vi "Read Text_File_PWL.vi"(8 "error in (no error)":errorcluster caption="에러 입력(에러 없음)", 11 "Text File 입력":refnum<class "Text File.lvclass">) -> (0 "error out":errorcluster caption="에러 출력", 2 "Text_File_PWL":T1(array[cluster]) {"Frequency" min=40.0 max=300.0 step=1.0; "Cycle" items=["0.5"=0.5, "1"=1.0, "1.5"=1.5, "2"=2.0, "2.5"=2.5, "3"=3.0, "3.5"=3.5, "4"=4.0, "4.5"=4.5, "5"=5.0, "5.5"=5.5, "6"=6.0, "6.5"=6.5, "7"=7.0, "7.5"=7.5, "8"=8.0, "8.5"=8.5, "9"=9.0, "9.5"=9.5, "10"=10.0, "10.5"=10.5, "11"=11.0, "11.5"=11.5, "12"=12.0, "12.5"=12.5, "13"=13.0, "13.5"=13.5, "14"=14.0, "14.5"=14.5, "15"=15.0, "15.5"=15.5, "16"=16.0, "16.5"=16.5, "17"=17.0, "17.5"=17.5, "18"=18.0, "18.5"=18.5, "19"=19.0, "19.5"=19.5, "20"=20.0, "20.5"=20.5, "21"=21.0, "21.5"=21.5, "22"=22.0, "22.5"=22.5, "23"=23.0, "23.5"=23.5, "24"=24.0, "24.5"=24.5, "25"=25.0, "25.5"=25.5, "26"=26.0, "26.5"=26.5, "27"=27.0, "27.5"=27.5, "28"=28.0, "28.5"=28.5, "29"=29.0, "29.5"=29.5, "30"=30.0, "30.5"=30.5, "31"=31.0, "31.5"=31.5, "32"=32.0, "32.5"=32.5, "33"=33.0, "33.5"=33.5, "34"=34.0, "34.5"=34.5, "35"=35.0, "35.5"=35.5, "36"=36.0, "36.5"=36.5, "37"=37.0, "37.5"=37.5, "38"=38.0, "38.5"=38.5, "39"=39.0, "39.5"=39.5, "40"=40.0, "40.5"=40.5, "41"=41.0, "41.5"=41.5, "42"=42.0, "42.5"=42.5, "43"=43.0, "43.5"=43.5, "44"=44.0, "44.5"=44.5, "45"=45.0, "45.5"=45.5, "46"=46.0, "46.5"=46.5, "47"=47.0, "47.5"=47.5, "48"=48.0, "48.5"=48.5, "49"=49.0, "49.5"=49.5, "50"=50.0, "50.5"=50.5, "51"=51.0, "51.5"=51.5, "52"=52.0, "52.5"=52.5, "53"=53.0, "53.5"=53.5, "54"=54.0, "54.5"=54.5, "55"=55.0, "55.5"=55.5, "56"=56.0, "56.5"=56.5, "57"=57.0, "57.5"=57.5, "58"=58.0, "58.5"=58.5, "59"=59.0, "59.5"=59.5, "60"=60.0, "60.5"=60.5, "61"=61.0, "61.5"=61.5, "62"=62.0, "62.5"=62.5, "63"=63.0, "63.5"=63.5, "64"=64.0, "64.5"=64.5, "65"=65.0, "65.5"=65.5, "66"=66.0, "66.5"=66.5, "67"=67.0, "67.5"=67.5, "68"=68.0, "68.5"=68.5, "69"=69.0, "69.5"=69.5, "70"=70.0, "70.5"=70.5, "71"=71.0, "71.5"=71.5, "72"=72.0, "72.5"=72.5, "73"=73.0, "73.5"=73.5, "74"=74.0, "74.5"=74.5, "75"=75.0, "75.5"=75.5, "76"=76.0, "76.5"=76.5, "77"=77.0, "77.5"=77.5, "78"=78.0, "78.5"=78.5, "79"=79.0, "79.5"=79.5, "80"=80.0, "80.5"=80.5, "81"=81.0, "81.5"=81.5, "82"=82.0, "82.5"=82.5, "83"=83.0, "83.5"=83.5, "84"=84.0, "84.5"=84.5, "85"=85.0, "85.5"=85.5, "86"=86.0, "86.5"=86.5, "87"=87.0, "87.5"=87.5, "88"=88.0, "88.5"=88.5, "89"=89.0, "89.5"=89.5, "90"=90.0, "90.5"=90.5, "91"=91.0, "91.5"=91.5, "92"=92.0, "92.5"=92.5, "93"=93.0, "93.5"=93.5, "94"=94.0, "94.5"=94.5, "95"=95.0, "95.5"=95.5, "96"=96.0, "96.5"=96.5, "97"=97.0, "97.5"=97.5, "98"=98.0, "98.5"=98.5, "99"=99.0, "99.5"=99.5, "100"=100.0, "100.5"=100.5, "101"=101.0, "101.5"=101.5, "102"=102.0, "102.5"=102.5, "103"=103.0, "103.5"=103.5, "104"=104.0, "104.5"=104.5, "105"=105.0, "105.5"=105.5, "106"=106.0, "106.5"=106.5, "107"=107.0, "107.5"=107.5, "108"=108.0, "108.5"=108.5, "109"=109.0, "109.5"=109.5, "110"=110.0, "110.5"=110.5, "111"=111.0, "111.5"=111.5, "112"=112.0, "112.5"=112.5, "113"=113.0, "113.5"=113.5, "114"=114.0, "114.5"=114.5, "115"=115.0, "115.5"=115.5, "116"=116.0, "116.5"=116.5, "117"=117.0, "117.5"=117.5, "118"=118.0, "118.5"=118.5, "119"=119.0, "119.5"=119.5, "120"=120.0, "120.5"=120.5, "121"=121.0, "121.5"=121.5, "122"=122.0, "122.5"=122.5, "123"=123.0, "123.5"=123.5, "124"=124.0, "124.5"=124.5, "125"=125.0, "125.5"=125.5, "126"=126.0, "126.5"=126.5, "127"=127.0, "127.5"=127.5]; "Amplitude" items=["0"=0.0, "10"=0.1, "20"=0.2, "30"=0.3, "40"=0.4, "50"=0.5, "60"=0.6, "70"=0.7, "80"=0.8, "90"=0.9, "100"=1.0]; "Ramp" items=["Step"=0, "Ramp (Lin.)"=2, "Ramp (Exp.)"=3]; "Shape" items=["Sine", "Square"]}, 3 "Text File 출력":refnum<class "Text File.lvclass">)   [LabVIEW 2020, in "Text File.lvclass"]
uses:
  Text File.lvclass
  Text File.lvclass/Text File.ctl
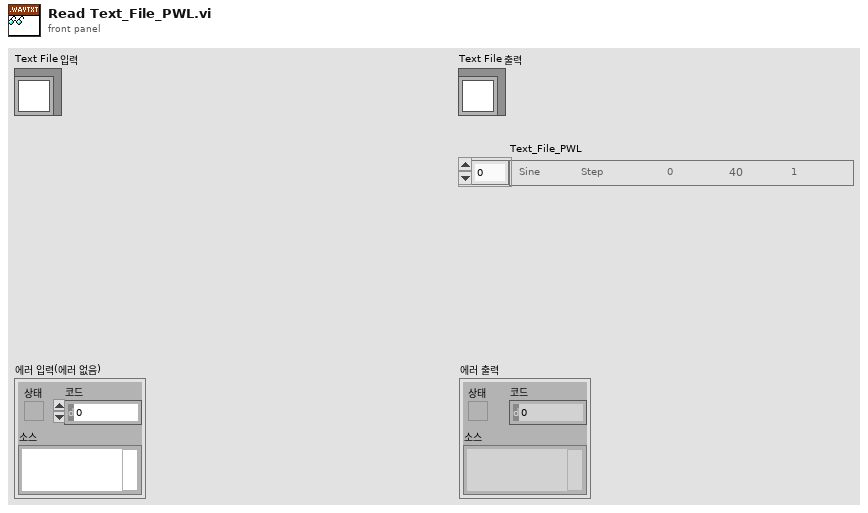
[diagram p1: front panel]
types:
  T1 = cluster{"Shape":u16, "Ramp":u16, "Amplitude":dbl, "Frequency":dbl, "Cycle":dbl}[]
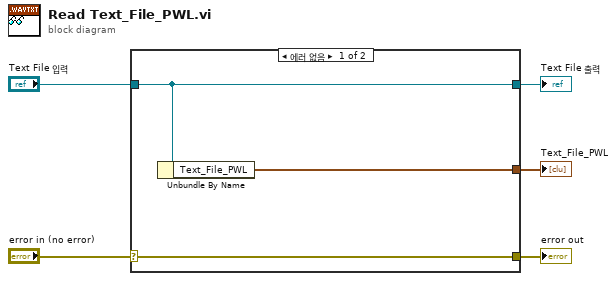
[diagram p0: block diagram]
diagram:
  n1 = case shown="에러 없음" "error in (no error)" {
    selector: "error in (no error)" -> [w8 w9]
    tunnel: [w8 w9] -> w4
    tunnel: [w7 w10] -> w2
    tunnel: "Text File 입력" -> [w7 w10]
    tunnel: [w6 _] -> w1
    frame No Error {
      n2 = Unbundle By Name(w7) -> ("Text_File_PWL"=w6:T1)
    }
    frame Error {
    }
  }
  "error out" <- w4
  "Text File 출력" <- w2
  "Text_File_PWL" <- w1
